vi "test Abort Copy Blob.vi"(8 "error in (no error)":errorcluster, 11 "TestCase in":refnum<class "Test_Blob.lvclass">) -> (0 "error out":errorcluster, 3 "TestCase out":refnum<class "Test_Blob.lvclass">)   [LabVIEW 2015, in "Test_Blob.lvclass"]
uses:
  Test_Blob.lvclass
  Blob Storage/Blob Type.ctl
  Global Parameters.vi
  Core/Session/Session.lvclass
  Blob Storage/NI_Azure_Blob.lvlib
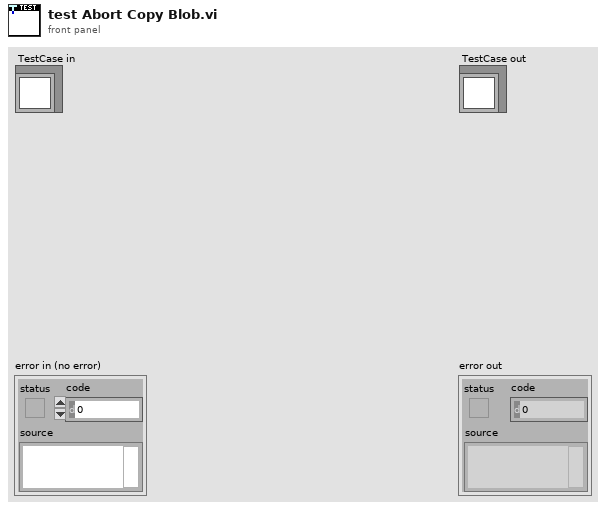
[diagram p1: front panel]
types:
  T1 = typedef "NI_Azure_Blob.lvlib/Blob Type.ctl" = enum16{"BlockBlob", "PageBlob", "AppendBlob"}
  T2 = typedef "NI_Azure_Core.lvlib/Session.lvclass/Azure Credentials.ctl" = cluster{"Storage Account Name":string, "Access Key":string}
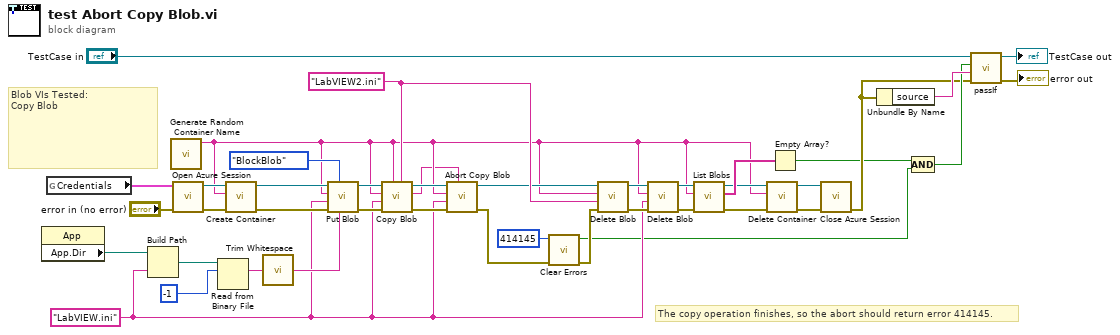
[diagram p0: block diagram]
diagram:
  w10 = "LabVIEW2.ini"
  w5 = "LabVIEW.ini"
  # "The copy operation finishes, so the abort should return error 414145."
  # "Blob VIs Tested:\nCopy Blob"
  n1 = property class="App"() -> ("App.Dir"=w37:path)  [unwired: 2 in, 2 out]
  n2 = global read "Global Parameters.vi" "Credentials"() -> (w21:T2)
  n3 = Build Path(base path=w37, name or relative path=w5) -> (appended path=w36:path)
  n4 = call "Generate Random Container Name.vi"() -> ("Random Container Name"=w6:string)  [unwired: 11 in]
  n5 = call "Open Azure Session.vi"("error in (no error)"="error in (no error)", "Credentials"=w21) -> ("error out"=w22:errorcluster, "Azure Session"=w18:refnum<class "Session.lvclass">)  [unwired: 8 in]
  n6 = Read from Binary File(10:-1 ("count (1)"), 11:w36) -> (2:w30:string)  [unwired: 4 in, 3 out]
  n7 = call "Create Container.vi"("error in (no error)"=w22, "Container"=w6, "Azure Session in"=w18) -> ("error out"=w34:errorcluster, "Azure Session out"=w33:refnum<class "Session.lvclass">)  [unwired: 7 in]
  n8 = call <vilib>:"Trim Whitespace.vi"("string"=w30) -> ("trimmed string"=w14:string)  [unwired: 1 in]
  n9 = call "Put Blob.vi"("Blob Content"=w14, "Blob type"=Blob_Type."BlockBlob", "error in (no error)"=w34, "Blob"=w5, "Container"=w6, "Azure Session in"=w33) -> ("error out"=w32:errorcluster, "Azure Session out"=w31:refnum<class "Session.lvclass">)  [unwired: 4 in]
  n10 = call "Copy Blob.vi"("Destination Blob"=w10, "Destination Container"=w6, "error in (no error)"=w32, "Source Blob"=w5, "Source Container"=w6, "Azure Session in"=w31) -> ("error out"=w29:errorcluster, "Copy ID"=w4:string, "Azure Session out"=w8:refnum<class "Session.lvclass">)  [unwired: 3 in]
  n11 = call "Abort Copy Blob.vi"("Copy ID"=w4, "error in (no error)"=w29, "Blob"=w5, "Container"=w6, "Azure Session in"=w8) -> ("error out"=w9:errorcluster, "Azure Session out"=w7:refnum<class "Session.lvclass">)  [unwired: 5 in]
  n12 = call <vilib>:"Clear Errors.vi"("error in (no error)"=w9, "specific error code to clear (0: all)"=414145) -> ("error out"=w3:errorcluster, "specific error cleared?"=w1:bool)  [unwired: 4 in]
  n13 = call "Delete Blob.vi"("error in (no error)"=w3, "Blob"=w10, "Container"=w6, "Azure Session in"=w7) -> ("error out"=w12:errorcluster, "Azure Session out"=w11:refnum<class "Session.lvclass">)  [unwired: 6 in]
  n14 = call "Delete Blob.vi"("error in (no error)"=w12, "Blob"=w5, "Container"=w6, "Azure Session in"=w11) -> ("error out"=w28:errorcluster, "Azure Session out"=w27:refnum<class "Session.lvclass">)  [unwired: 6 in]
  n15 = call "List Blobs.vi"("error in (no error)"=w28, "Container"=w6, "Azure Session in"=w27) -> ("error out"=w25:errorcluster, "Blobs"=w26:string[], "Azure Session out"=w24:refnum<class "Session.lvclass">)  [unwired: 6 in]
  n16 = call "Delete Container.vi"("error in (no error)"=w25, "Container"=w6, "Azure Session in"=w24) -> ("error out"=w20:errorcluster, "Azure Session out"=w15:refnum<class "Session.lvclass">)  [unwired: 7 in]
  n17 = Empty Array?(array=w26) -> (empty?=w13:bool)
  n18 = call "Close Azure Session.vi"("error in (no error)"=w20, "Azure Session"=w15) -> ("error out"=w16:errorcluster)  [unwired: 9 in]
  n19 = Unbundle By Name(w16) -> ("source"=w38:string)
  n20 = Compound Arithmetic op=AND(w13, w1) -> (w19:bool)
  n21 = call-dynamic "passIf.vi"("error in (no error)"=w16, "message (\"\")"=w38, "pass"=w19, "TestCase in"="TestCase in") -> ("error out"=→"error out":errorcluster, "TestCase out"=→"TestCase out":refnum<class "Test_Blob.lvclass">)  [unwired: 6 in]
